vi "EOL.vi"() -> (3 "eol":string)   [LabVIEW 2020, in "infolib.lvlib"]
doc: "Returns end of line according conditional symbols in project settings."
uses:
  infolib.lvlib
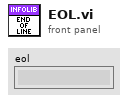
[diagram p1: front panel]
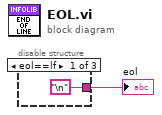
[diagram p0: block diagram]
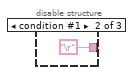
[diagram p2: hidden frame]
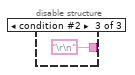
[diagram p3: hidden frame]
diagram:
  n1 = disable-structure shown="eol==lf" {
    disable-tunnel: ["\n" "\r" "\r\n"] -> w1
    frame condition #0 (active) {
    }
    frame condition #1 {
    }
    frame condition #2 {
    }
  }
  "eol" <- w1
